vi "txtFileRead.vi"(11 "file path (dialog if empty)":path caption="文件路径 （空时为对话框）") -> (3 "all rows":string[][](array[string]))   [LabVIEW 2011]
uses:
  <vilib>/Utility/file.llb/Read From Spreadsheet File (string).vi
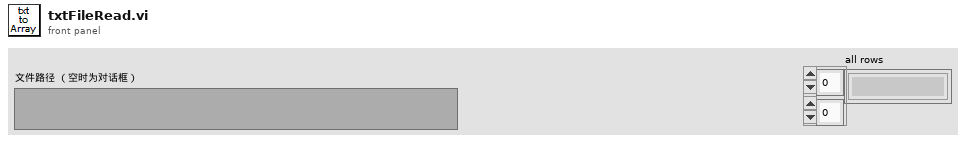
[diagram p1: front panel]
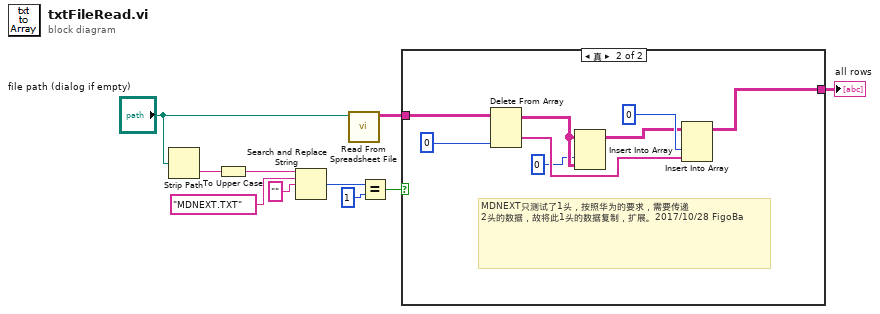
[diagram p0: block diagram]
diagram:
  n1 = Strip Path(path="file path (dialog if empty)") -> (name=w10:string)  [unwired: 1 out]
  n2 = To Upper Case(1:w10) -> (0:w9:string)
  n3 = Search and Replace String(input string=w9, search string="MDNEXT.TXT" ("搜索字符串"), replace string="" ("替换字符串(\"\")")) -> (number of replacements=w6:i32)  [unwired: 5 in, 3 out]
  n4 = call-poly <vilib>:"Read From Spreadsheet File.vi"("file path (dialog if empty)"="file path (dialog if empty)") -> ("all rows"=w3:string[][])  [unwired: 6 in, 4 out]
  n5 = Equal?(x=w6, y=1) -> (x = y?=w4:bool)
  n6 = case shown="真" w4 {
    tunnel: w3 -> [w11 w19]
    tunnel: [w11 w12] -> w1
    frame False {
    }
    frame True {
      # "MDNEXT只测试了1头，按照华为的要求，需要传递\n2头的数据，故将此1头的数据复制，扩展。2017/10/28 FigoBa"
      n7 = Delete From Array(array=w19, index (col)=0 ("禁用的索引 (列)")) -> (deleted portion=w17:string[], array with subset deleted=w15:string[][])  [unwired: 2 in]
      n8 = Insert Into Array(array=w15, index (col)=0 ("禁用的索引 (列)"), new element=w15) -> (w13:string[][])  [unwired: 1 in]
      n9 = Insert Into Array(array=w13, index (col)=0 ("禁用的索引 (列)"), new element=w17) -> (w12:string[][])  [unwired: 1 in]
    }
  }
  "all rows" <- w1
